vi "CgInit.vi"(5 "Sampling Frequency (0)":u32, 6 "error in (no error)":errorcluster, 8 "Calibration File":path, 9 "VISA resource name":refnum<visa-resource-name>) -> (0 "error out":errorcluster, 1 "Sensor Names":string[](array[string]), 2 "#Sensors":i32, 3 "VISA resource name out":refnum<visa-resource-name>, 4 "Calibration Array":cluster{"Offset":dbl, "Gain":dbl}[](array[cluster]))   [LabVIEW 2012]
doc: "Initializes the cyberglove for use in the experiment.\n\nSets up a certain sampling rate on the glove, changes button and light behavior, creates a custom censor of sensors. Additionally, extracts information about the cyberglove, such as the the sensor names.\n\nLoads a calibration file and aligns it with the current senosrs to produce a calibration array for use in interpretting the data."
uses:
  <vilib>/Instr/_visa.llb/Select Event Type.ctl
  <vilib>/Instr/_visa.llb/VISA Configure Serial Port (Instr).vi
  GlobalVariables.vi
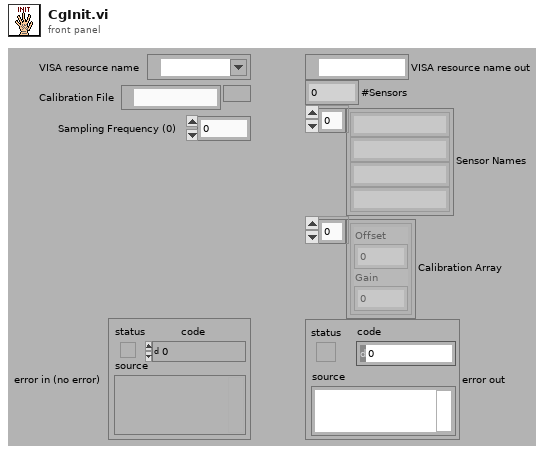
[diagram p1: front panel]
types:
  T1 = typedef "Select Event Type.ctl" = u32
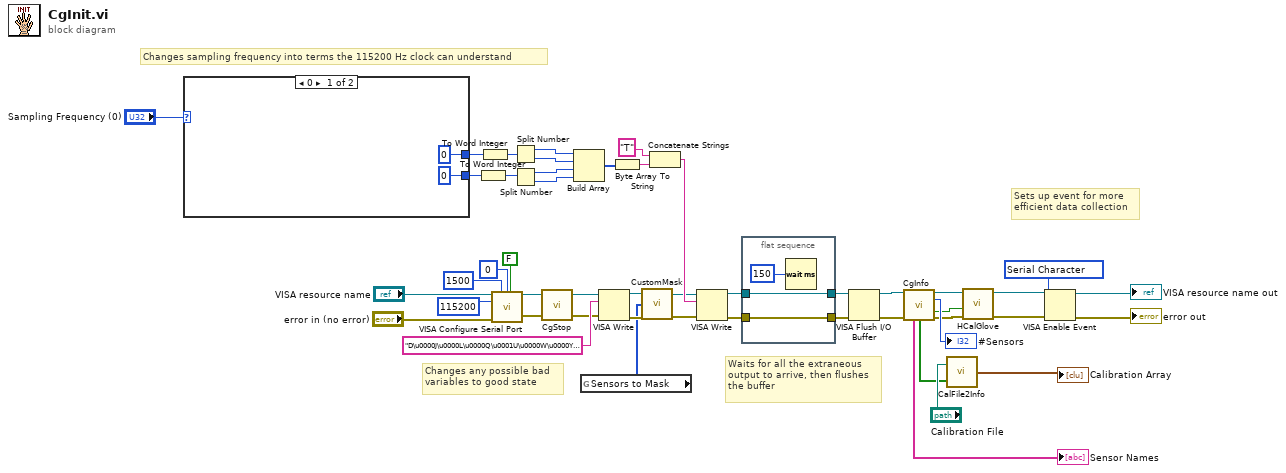
[diagram p0: block diagram]
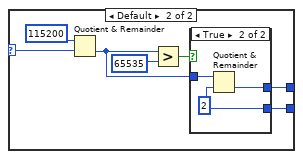
[diagram p2: hidden frame]
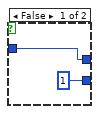
[diagram p3: hidden frame]
diagram:
  w1 = T1 1073684533 items=["Service Request"=1073684491, "Trigger"=3221168138, "Clear"=1073684493, "VXI Signal"=1073684512, "VXI/VME Interrupt"=3221168161, "VXI/VME Sysfail"=1073684509, "VXI/VME Sysreset"=1073684510, "GPIB CIC"=1073684498, "GPIB Talk"=1073684499, "GPIB Listen"=1073684500, "PXI Interrupt"=1073684514, "Serial Break"=1073684515, "Serial TermChar"=1073684516, "Serial CTS"=1073684521, "Serial DSR"=1073684522, "Serial DCD"=1073684524, "Serial RI"=1073684526, "Serial Character"=1073684533, "USB Interrupt"=1073684535, "All Enabled"=1073709055] ("Event Type")
  # "Sets up event for more\nefficient data collection"
  # "Changes sampling frequency into terms the 115200 Hz clock can understand"
  # "Waits for all the extraneous\noutput to arrive, then flushes\nthe buffer"
  # "Changes any possible bad\nvariables to good state"
  n1 = case shown="0" "Sampling Frequency (0)" {
    selector: "Sampling Frequency (0)" -> [_ w51]
    tunnel: [u32 0 w53] -> w34
    tunnel: [u32 0 ("y") w52] -> w35
    frame 0 {
    }
    frame Default {
      n2 = Quotient & Remainder(x=u32 115200, y=w51) -> (floor(x/y)=w54:u32)  [unwired: 1 out]
      n3 = Greater?(x=w54, y=u32 65535) -> (0:w55:bool)
      n4 = case shown="True" w55 {
        tunnel: w54 -> [w59 w62]
        tunnel: [w59 w61] -> w53
        tunnel: [u32 1 ("y") w60] -> w52
        frame False {
        }
        frame True {
          w60 = u32 2 ("y")
          n5 = Quotient & Remainder(x=w62, y=w60) -> (floor(x/y)=w61:u32)  [unwired: 1 out]
        }
      }
    }
  }
  n6 = To Word Integer(number=w35) -> (16bit integer=w33:i16)
  n7 = To Word Integer(number=w34) -> (16bit integer=w32:i16)
  n8 = call-poly "VISA Configure Serial Port"("VISA resource name"="VISA resource name", "timeout (10sec)"=u32 1500, "termination char\n(0xA = '\\n' = LF)"=u8 0 ("termination char\n(0xA = '\\n' = LF)"), "Enable Termination\nChar (T)"=FALSE ("Enable Termination\nChar (T)"), "baud rate (9600)"=u32 115200, "error in (no error)"="error in (no error)") -> ("VISA resource name out"=w20:refnum<visa-resource-name>, "error out"=w19:errorcluster)  [unwired: 8 in]
  n9 = Split Number(x=w32) -> (hi(x)=w31:u8, lo(x)=w30:u8)
  n10 = Split Number(x=w33) -> (hi(x)=w29:u8, lo(x)=w28:u8)
  n11 = call "CgStop.vi"("error in (no error)"=w19, "VISA resource name"=w20) -> ("error out"=w15:errorcluster, "VISA resource name out"=w14:refnum<visa-resource-name>)  [unwired: 2 in]
  n12 = Build Array(w31, w30, w29, w28) -> (w27:u8[])
  n13 = global read "GlobalVariables.vi" "Sensors to Mask"() -> (w2:u32[])
  n14 = VISA Write(VISA resource name=w14, write buffer="D\u0000J\u0000L\u0000Q\u0001U\u0000W\u0000Y\u0000", error in (no error)=w15) -> (VISA resource name out=w13:refnum<visa-resource-name>, error out=w12:errorcluster)  [unwired: 1 out]
  n15 = Byte Array To String(unsigned byte array=w27) -> (string=w25:string)
  n16 = call "CustomMask.vi"("error in (no error)"=w12, "Custom Mask"=w2, "VISA resource name"=w13) -> ("error out"=w21:errorcluster, "VISA resource name out"=w22:refnum<visa-resource-name>)
  n17 = Concatenate Strings("T" ("string"), w25) -> (w24:string)
  n18 = VISA Write(VISA resource name=w22, write buffer=w24, error in (no error)=w21) -> (VISA resource name out=w11:refnum<visa-resource-name>, error out=w10:errorcluster)  [unwired: 1 out]
  n19 = flat-sequence {
    tunnel: w11 -> [w65]
    tunnel: [w65] -> w17
    tunnel: w10 -> [w64]
    tunnel: [w64] -> w16
    frame #0 {
      n20 = Wait (ms)(milliseconds to wait=u32 150) -> ()  [unwired: 1 out]
    }
  }
  n21 = VISA Flush I/O Buffer(VISA resource name=w17, error in (no error)=w16) -> (VISA resource name out=w9:refnum<visa-resource-name>, error out=w8:errorcluster)  [unwired: 1 in]
  n22 = call "CgInfo.vi"("VISA resource name"=w9, "error in (no error)"=w8) -> ("VISA resource name out"=w7:refnum<visa-resource-name>, "#Sensors"=→"#Sensors":i32, "RH?"=w5:bool, "Sensor Names"=→"Sensor Names":string[], "Sensors Active"=w45:bool[], "error out"=w6:errorcluster)  [unwired: 7 in, 1 out]
  n23 = call "CalFile2Info.vi"("Calibration File"="Calibration File", "Sensors Active"=w45) -> ("Calibration Array"=→"Calibration Array":cluster{"Offset":dbl, "Gain":dbl}[])  [unwired: 2 in]
  n24 = call "HCalGlove.vi"("error in (no error)"=w6, "RH?"=w5, "VISA Resource In"=w7) -> ("error out"=w3:errorcluster, "VISA Resource Out"=w4:refnum<visa-resource-name>)  [unwired: 2 in, 1 out]
  n25 = VISA Enable Event(8:w3, 10:w1, 11:w4) -> (0:→"error out":errorcluster, 3:→"VISA resource name out":refnum<visa-resource-name>)  [unwired: 1 in]
